vi "PopupWebBrowerHelp.vi"(11 "File Path IN":path) -> ()   [LabVIEW 2010]
uses:
  030 - EVENTS/EnumFgvEventCommand.ctl
  090 - ERRORS/Ctrls/enumLogAndView.ctl
  020 - HMI/SubVis/enumDeferPanelUpdate.ctl
  030 - EVENTS/02 - ToScreens/ToScreensCommand.ctl
panel:
  out "Logo 600 X 200":picture
  in  "StringParam":string
  in  "WebBrowser":refnum<k7>(container)
  in  "bouton_quitter":bool
  # "Aide en ligne"
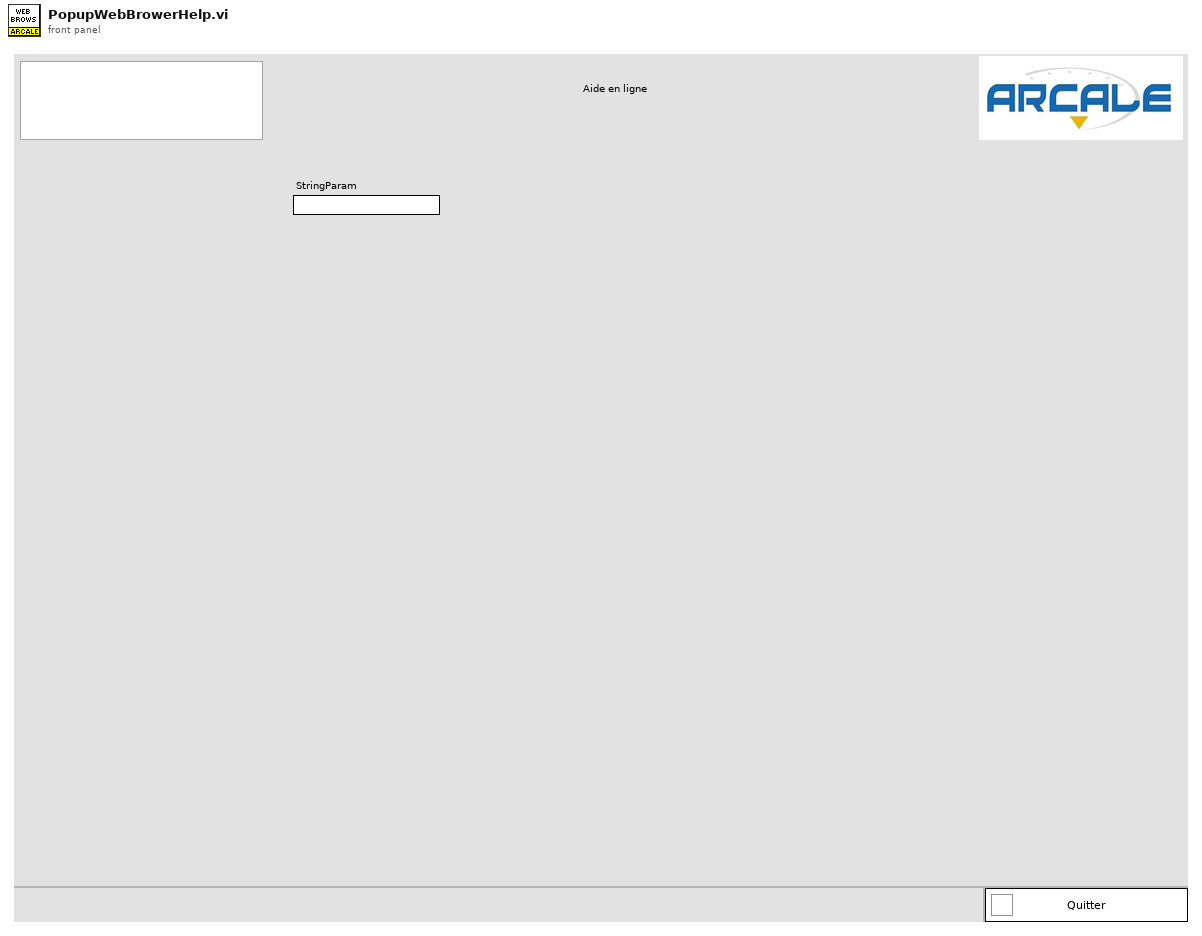
[diagram p1: front panel]
types:
  T1 = typedef "enumLogAndView.ctl" = enum16{"Log only", "Log and view"}
  T2 = typedef "EnumFgvEventCommand.ctl" = enum16{"Setup", "Cleanup", "Get"}
  T3 = typedef "enumDeferPanelUpdate.ctl" = enum16{"suspend layout", "resume layout"}
  T4 = typedef "ToScreensCommand.ctl" = enum16{"Stop screen", "Stop all screens"}
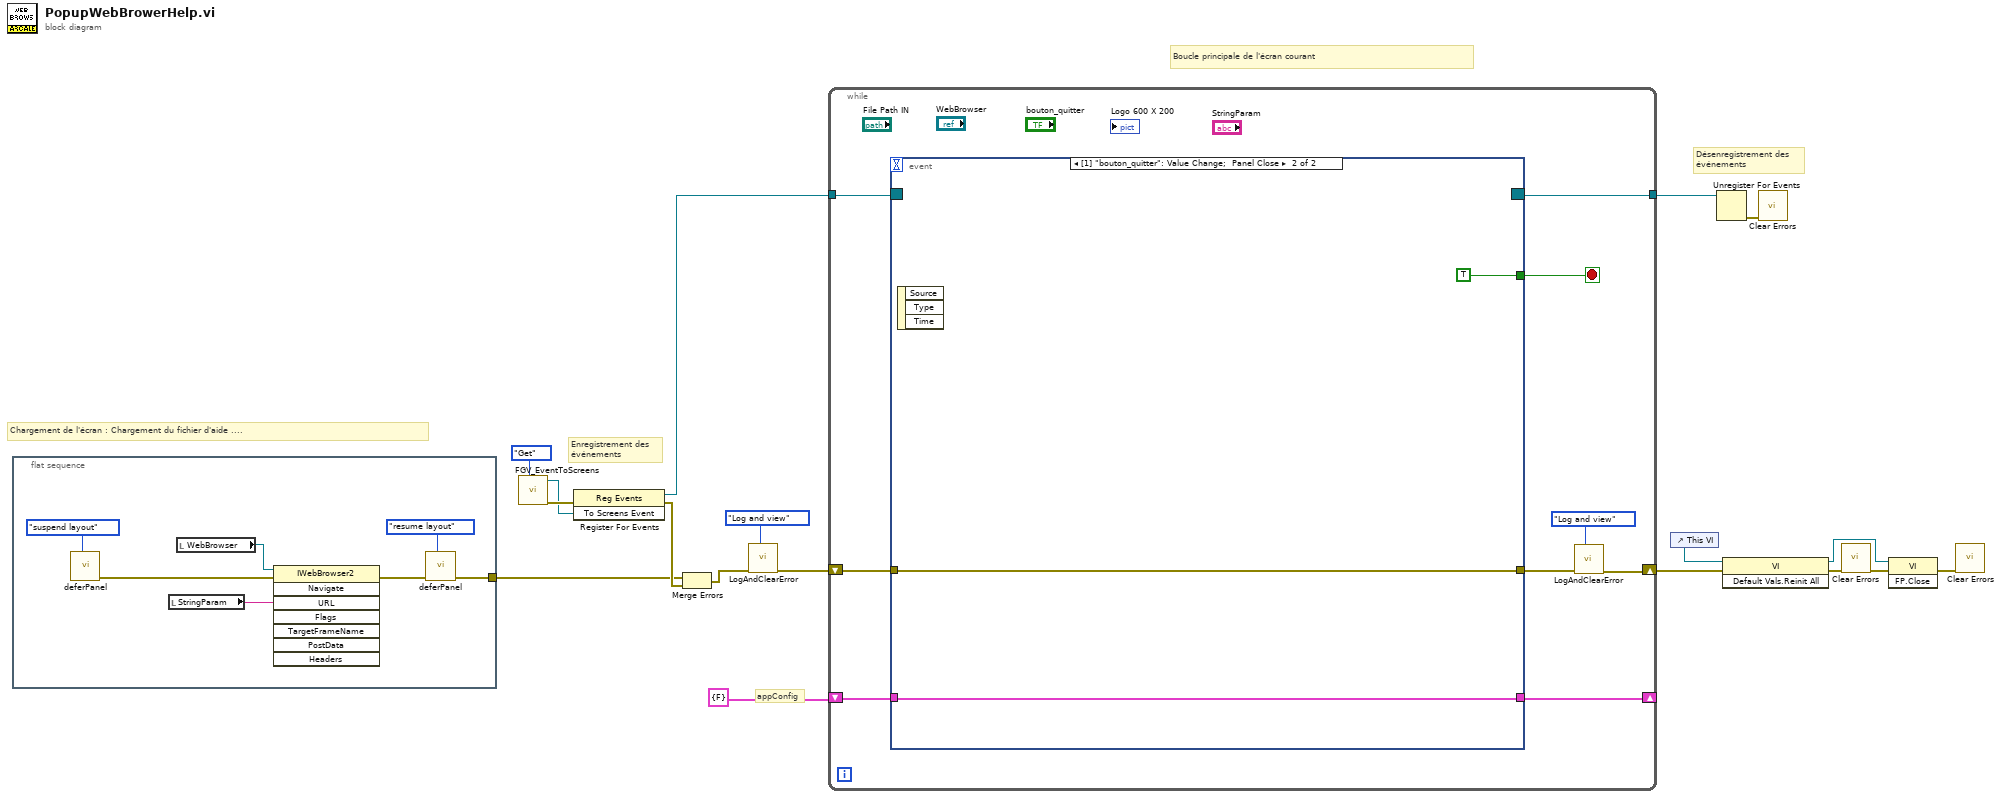
[diagram p0: block diagram]
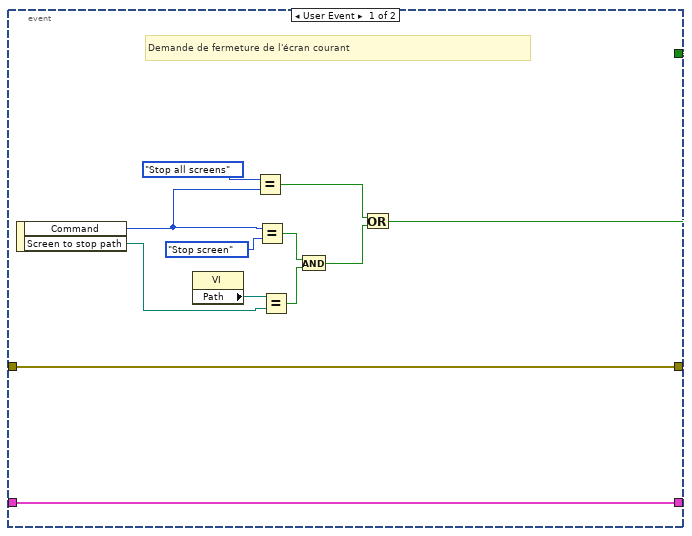
[diagram p2: hidden frame]
diagram:
  # "Chargement de l'écran : Chargement du fichier d'aide ...."
  # "Boucle principale de l'écran courant"
  # "appConfig"
  # "Désenregistrement des \névénements"
  # "Enregistrement des \névénements"
  n1 = flat-sequence {
    tunnel: [w19] -> w1
    frame #0 {
      n2 = call "deferPanel.vi"("EnumDeferPanel"=enumDeferPanelUpdate."suspend layout") -> ("error out"=w25:errorcluster)  [unwired: 2 in, 8 out]
      n3 = local read "StringParam"() -> (w20:string)
      n4 = local read "WebBrowser"() -> (w21:refnum<k7>)
      n5 = invoke class="IWebBrowser2" method="Navigate"(reference=w21, error in=w25, "URL"=w20) -> (error out=w24:errorcluster)  [unwired: 5 in, 7 out]
      n6 = call "deferPanel.vi"("EnumDeferPanel"=enumDeferPanelUpdate."resume layout", "errorIn"=w24) -> ("error out"=w19:errorcluster)  [unwired: 1 in, 8 out]
    }
  }
  n7 = call "FGV_EventToScreens.vi"("Command"=EnumFgvEventCommand."Get") -> ("error out"=w18:errorcluster, "To Screens Event"=w17:refnum<user-event>)  [unwired: 9 in]
  n8 = register-events(error in=w18, w17) -> (reference out=w16:refnum<event-registration>, error out=w8:errorcluster)  [unwired: 1 in]
  n9 = Merge Errors(w1, w8) -> (w6:errorcluster)
  n10 = call "LogAndClearError.vi"("Log and view ?"=enumLogAndView."Log and view", "error in (no error)"=w6) -> ("error out"=w5:errorcluster)  [unwired: 9 in]
  n11 = while {
    tunnel: w16 -> [w34]
    shift-right: [w27] -> w9
    shift-left: w5 -> [w33]
    tunnel: [w32] -> w15
    shift-right: [w30] -> _
    shift-left: cluster{"Boolean":bool} {"Boolean"=FALSE} ("appConfig") -> [w31]
    stop <- w29 stop-if-true
    n12 = event shown="[1] \"bouton_quitter\": Value Change;  Panel Close" {
      selector: w34 -> [_ _]
      dyn-events: [_ _] -> w32
      timeout: _ -> [_ _]
      tunnel: [w35 TRUE ("stopCurrentScreen")] -> w29
      tunnel: w33 -> [w45 w47]
      tunnel: [w45 w47] -> w28
      tunnel: w31 -> [w46 w48]
      tunnel: [w46 w48] -> w30
      event User Event {
        # "Demande de fermeture de l'écran courant"
        n13 = event-data() -> ("Command"=w43:T4, "Screen to stop path"=w40:path)  [unwired: 1 out]
        n14 = property class="VI"() -> ("Path"=w41:path)  [unwired: 2 in, 2 out]
        n15 = Equal?(x=ToScreensCommand."Stop all screens", y=w43) -> (x = y?=w37:bool)
        n16 = Equal?(x=w43, y=ToScreensCommand."Stop screen") -> (x = y?=w39:bool)
        n17 = Equal?(x=w41, y=w40) -> (x = y?=w38:bool)
        n18 = And(x=w39, y=w38) -> (x .and. y?=w36:bool)
        n19 = Or(x=w37, y=w36) -> (x .or. y?=w35:bool)
      }
      event "bouton_quitter": Value Change; Panel Close {
        n20 = event-data() -> ()  [unwired: 4 out]
      }
    }
    n21 = call "LogAndClearError.vi"("Log and view ?"=enumLogAndView."Log and view", "error in (no error)"=w28) -> ("error out"=w27:errorcluster)  [unwired: 9 in]
  }
  n22 = control-ref of="This VI"() -> (w12:refnum<vi>)
  n23 = Unregister For Events(event registration refnum=w15) -> (error out=w13:errorcluster)  [unwired: 1 in]
  n24 = invoke class="VI" method="Default Vals.Reinit All"(reference=w12, error in=w9) -> (reference out=w2:refnum<vi>, error out=w11:errorcluster)  [unwired: 1 in, 1 out]
  n25 = call <vilib>:"Clear Errors.vi"("error in (no error)"=w13) -> ()  [unwired: 7 out]
  n26 = call <vilib>:"Clear Errors.vi"("error in (no error)"=w11) -> ("error out"=w3:errorcluster)  [unwired: 6 out]
  n27 = invoke class="VI" method="FP.Close"(reference=w2, error in=w3) -> (error out=w4:errorcluster)  [unwired: 1 in, 2 out]
  n28 = call <vilib>:"Clear Errors.vi"("error in (no error)"=w4) -> ()  [unwired: 7 out]
